vi "Finish.vi"   [LabVIEW 2020]
doc: "This VI is called just before exiting. It is expected to close I/O refnum, save collected data, etc."
uses:
  <vilib>/Rock Robotics/WPI/Utilities/WPI_GetSetVariantRefNum.vi
types:
  T1 = typedef "WPI_DigitalOutputDevRef.ctl" = cluster{"DIO Channel":T2, "DevStatus":errorcluster}
  T2 = typedef "FPGA_DIOChannel.ctl" = enum8{"DIO 0", "DIO 1", "DIO 2", "DIO 3", "DIO 4", "DIO 5", "DIO 6", "DIO 7", "DIO 8", "DIO 9", "DIO MXP 0", "DIO MXP 1", "DIO MXP 2", "DIO MXP 3", "DIO MXP 4", "DIO MXP 5", "DIO MXP 6", "DIO MXP 7", "DIO MXP 8", "DIO MXP 9", "DIO MXP 10", "DIO MXP 11", "DIO MXP 12", "DIO MXP 13", "DIO MXP 14", "DIO MXP 15", "SPI Port CS1", "SPI Port CS2", "SPI Port CS3", "SPI Port MISO", "SPI Port MOSI", "Invalid"}
  T3 = typedef "WPI_MotorControlDeviceRef.ctl" = cluster{"DeviceStatus":errorcluster, "Type":T4, "PWM":cluster{"PWM Channel":T5, "DeadBand":T6}, "CAN":cluster{"Device Number":u8, "SetOutput VI Ref":variant, "GetOutput VI Ref":variant, "Enable VI Ref":variant, "Disable VI Ref":variant, "Data":variant}, "Invert":bool, "DIO PWM":cluster{"PWM \"Enable\" Channel":T5, "DIOChannel":T2, "PWM Rate":dbl}}
  T4 = typedef "WPI_MotorControlType.ctl" = enum16{"PWM", "CAN", "DIO PWM"}
  T5 = typedef "FPGA_DIOPWMChannel.ctl" = enum8{"PWM 0", "PWM 1", "PWM 2", "PWM 3", "PWM 4", "PWM 5", "PWM 6", "PWM 7", "PWM 8", "PWM 9", "PWM MXP 0", "PWM MXP 1", "PWM MXP 2", "PWM MXP 3", "PWM MXP 4", "PWM MXP 5", "PWM MXP 6", "PWM MXP 7", "PWM MXP 8", "PWM MXP 9", "Invalid"}
  T6 = typedef "WPI_PWMDeadband.ctl" = cluster{"Name":string, "maxPositivePwm":i32, "minPositivePwm":i32, "centerPwm":i32, "maxNegativePwm":i32, "minNegativePwm":i32, "angularRange":u16}
  T7 = typedef "WPI_JoystickDevRef.ctl" = cluster{"Device":T8}
  T8 = typedef "WPI_JoystickDeviceEnum.ctl" = enum16{"USB 0", "USB 1", "USB 2", "USB 3", "USB 4", "USB 5"}
  T9 = typedef "WPI_SolenoidDevRef.ctl" = cluster{"DevStatus":errorcluster, "Pneumatics Control Module":u8, "Forward Solenoid Channel":T10, "Reverse Solenoid Channel":T10}
  T10 = typedef "WPI_SolenoidChannel.ctl" = enum8{"Solenoid 0", "Solenoid 1", "Solenoid 2", "Solenoid 3", "Solenoid 4", "Solenoid 5", "Solenoid 6", "Solenoid 7", "Solenoid 8", "Solenoid 9", "Solenoid 10", "Solenoid 11", "Solenoid 12", "Solenoid 13", "Solenoid 14", "Solenoid 15", "Invalid"}
  T11 = typedef "Color Sensor V3 DevRef.ctl" = cluster{"I2CDevRef":T12}
  T12 = typedef "WPI_I2CDevRef.ctl" = cluster{"DevStatus":errorcluster, "Device Address":u8, "Handle":i32, "I2C Bus":T13}
  T13 = typedef "i2c_bus.ctl" = enum16{"I2C On-Board", "I2C MXP", "Invalid"}
  T14 = typedef "WPI_SwitchDevRef.ctl" = cluster{"DevStatus":errorcluster, "DIO Channel":T2, "CntIndex":T15, "Normally Closed":bool}
  T15 = typedef "FPGA_CounterCtrSystemIndex.ctl" = enum8{"Ctr 0", "Ctr 1", "Ctr 2", "Ctr 3", "Ctr 4", "Ctr 5", "Ctr 6", "Ctr 7", "Invalid"}
  T16 = typedef "WPI_CompressorDevRef.ctl" = cluster{"DevStatus":errorcluster, "Pneumatics Control Module":u8}
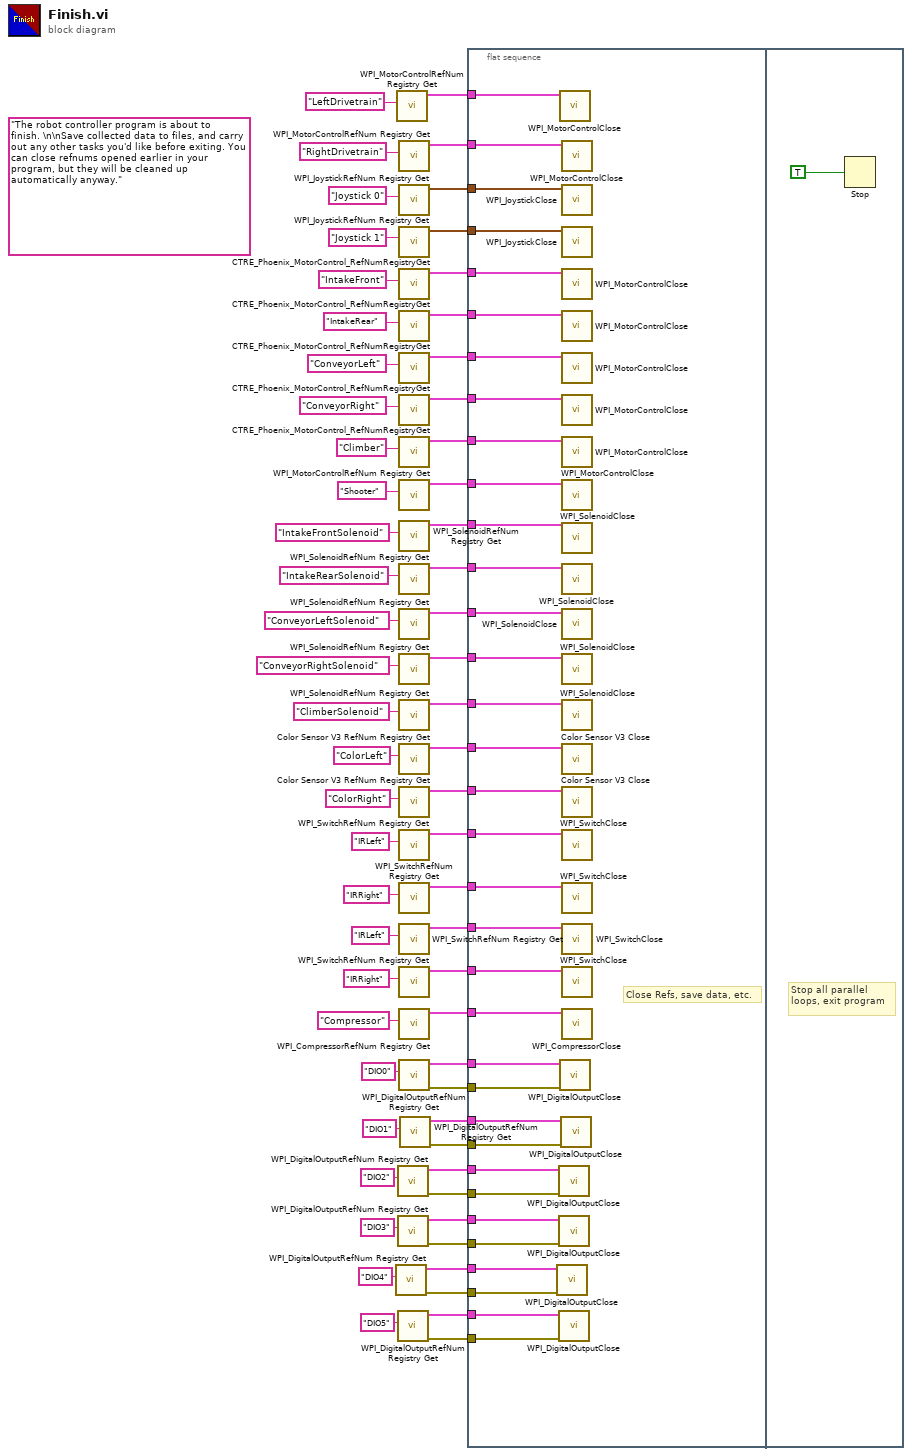
[diagram p0: block diagram]
diagram:
  (unwired) "The robot controller program is about to finish. \n\nSave collected data to files, and carry out any other tasks you'd like before exiting. You can close refnums opened earlier in your program, but they will be cleaned up automatically anyway."
  n1 = call <vilib>:"WPI_DigitalOutputRefNum Registry Get.vi"("refnum name"="DIO4") -> ("error out"=w11:errorcluster, "DigitalOutputDevRef"=w12:T1)  [unwired: 9 in]
  n2 = call <vilib>:"WPI_MotorControlRefNum Registry Get.vi"("refnum name"="LeftDrivetrain") -> ("MotorControlDevRef"=w24:T3)  [unwired: 9 in, 1 out]
  n3 = call <vilib>:"WPI_DigitalOutputRefNum Registry Get.vi"("refnum name"="DIO2") -> ("error out"=w14:errorcluster, "DigitalOutputDevRef"=w13:T1)  [unwired: 9 in]
  n4 = call <vilib>:"WPI_DigitalOutputRefNum Registry Get.vi"("refnum name"="DIO3") -> ("error out"=w8:errorcluster, "DigitalOutputDevRef"=w7:T1)  [unwired: 9 in]
  n5 = call <vilib>:"WPI_DigitalOutputRefNum Registry Get.vi"("refnum name"="DIO5") -> ("error out"=w5:errorcluster, "DigitalOutputDevRef"=w4:T1)  [unwired: 9 in]
  n6 = call <vilib>:"WPI_MotorControlRefNum Registry Get.vi"("refnum name"="RightDrivetrain") -> ("MotorControlDevRef"=w25:T3)  [unwired: 9 in, 1 out]
  n7 = call <vilib>:"WPI_JoystickRefNum Registry Get.vi"("refnum name"="Joystick 0") -> ("JoystickDevRef"=w61:T7)  [unwired: 1 in, 9 out]
  n8 = call <vilib>:"WPI_JoystickRefNum Registry Get.vi"("refnum name"="Joystick 1") -> ("JoystickDevRef"=w59:T7)  [unwired: 1 in, 9 out]
  n9 = call <vilib>:"CTRE_Phoenix_MotorControl_RefNumRegistryGet.vi"("refnum name"="IntakeFront") -> ("PhoenixMotorControlDevRef"=w58:T3)  [unwired: 9 in, 1 out]
  n10 = call <vilib>:"CTRE_Phoenix_MotorControl_RefNumRegistryGet.vi"("refnum name"="IntakeRear") -> ("PhoenixMotorControlDevRef"=w55:T3)  [unwired: 9 in, 1 out]
  n11 = call <vilib>:"CTRE_Phoenix_MotorControl_RefNumRegistryGet.vi"("refnum name"="ConveyorLeft") -> ("PhoenixMotorControlDevRef"=w51:T3)  [unwired: 9 in, 1 out]
  n12 = call <vilib>:"CTRE_Phoenix_MotorControl_RefNumRegistryGet.vi"("refnum name"="ConveyorRight") -> ("PhoenixMotorControlDevRef"=w50:T3)  [unwired: 9 in, 1 out]
  n13 = call <vilib>:"CTRE_Phoenix_MotorControl_RefNumRegistryGet.vi"("refnum name"="Climber") -> ("PhoenixMotorControlDevRef"=w49:T3)  [unwired: 9 in, 1 out]
  n14 = call <vilib>:"WPI_MotorControlRefNum Registry Get.vi"("refnum name"="Shooter") -> ("MotorControlDevRef"=w48:T3)  [unwired: 9 in, 1 out]
  n15 = call <vilib>:"WPI_SolenoidRefNum Registry Get.vi"("refnum name"="IntakeFrontSolenoid") -> ("SolenoidDevRef"=w43:T9)  [unwired: 9 in, 1 out]
  n16 = call <vilib>:"WPI_SolenoidRefNum Registry Get.vi"("refnum name"="IntakeRearSolenoid") -> ("SolenoidDevRef"=w33:T9)  [unwired: 9 in, 1 out]
  n17 = call <vilib>:"WPI_SolenoidRefNum Registry Get.vi"("refnum name"="ConveyorLeftSolenoid") -> ("SolenoidDevRef"=w42:T9)  [unwired: 9 in, 1 out]
  n18 = call <vilib>:"WPI_SolenoidRefNum Registry Get.vi"("refnum name"="ConveyorRightSolenoid") -> ("SolenoidDevRef"=w41:T9)  [unwired: 9 in, 1 out]
  n19 = call <vilib>:"WPI_SolenoidRefNum Registry Get.vi"("refnum name"="ClimberSolenoid") -> ("SolenoidDevRef"=w40:T9)  [unwired: 9 in, 1 out]
  n20 = call <vilib>:"Color Sensor V3 RefNum Registry Get.vi"("refnum name"="ColorLeft") -> ("ColorSensorDevRef"=w38:T11)  [unwired: 9 in, 1 out]
  n21 = call <vilib>:"Color Sensor V3 RefNum Registry Get.vi"("refnum name"="ColorRight") -> ("ColorSensorDevRef"=w37:T11)  [unwired: 9 in, 1 out]
  n22 = call <vilib>:"WPI_SwitchRefNum Registry Get.vi"("refnum name"="IRLeft") -> ("SwitchDevRef"=w32:T14)  [unwired: 9 in, 1 out]
  n23 = call <vilib>:"WPI_SwitchRefNum Registry Get.vi"("refnum name"="IRRight") -> ("SwitchDevRef"=w31:T14)  [unwired: 9 in, 1 out]
  n24 = call <vilib>:"WPI_SwitchRefNum Registry Get.vi"("refnum name"="IRLeft") -> ("SwitchDevRef"=w20:T14)  [unwired: 9 in, 1 out]
  n25 = call <vilib>:"WPI_SwitchRefNum Registry Get.vi"("refnum name"="IRRight") -> ("SwitchDevRef"=w19:T14)  [unwired: 9 in, 1 out]
  n26 = call <vilib>:"WPI_CompressorRefNum Registry Get.vi"("refnum name"="Compressor") -> ("CompressorDevRef"=w28:T16)  [unwired: 9 in, 1 out]
  n27 = call <vilib>:"WPI_DigitalOutputRefNum Registry Get.vi"("refnum name"="DIO0") -> ("error out"=w2:errorcluster, "DigitalOutputDevRef"=w1:T1)  [unwired: 9 in]
  n28 = call <vilib>:"WPI_DigitalOutputRefNum Registry Get.vi"("refnum name"="DIO1") -> ("error out"=w17:errorcluster, "DigitalOutputDevRef"=w18:T1)  [unwired: 9 in]
  n29 = flat-sequence {
    tunnel: w61 -> [w96]
    tunnel: w59 -> [w95]
    tunnel: w58 -> [w94]
    tunnel: w55 -> [w93]
    tunnel: w51 -> [w92]
    tunnel: w50 -> [w91]
    tunnel: w49 -> [w90]
    tunnel: w48 -> [w89]
    tunnel: w43 -> [w88]
    tunnel: w42 -> [w87]
    tunnel: w41 -> [w86]
    tunnel: w40 -> [w85]
    tunnel: w38 -> [w84]
    tunnel: w37 -> [w83]
    tunnel: w33 -> [w82]
    tunnel: w32 -> [w81]
    tunnel: w31 -> [w80]
    tunnel: w28 -> [w79]
    tunnel: w25 -> [w78]
    tunnel: w24 -> [w77]
    tunnel: w20 -> [w76]
    tunnel: w19 -> [w75]
    tunnel: w18 -> [w74]
    tunnel: w17 -> [w73]
    tunnel: w13 -> [w71]
    tunnel: w14 -> [w72]
    tunnel: w7 -> [w67]
    tunnel: w8 -> [w68]
    tunnel: w12 -> [w70]
    tunnel: w11 -> [w69]
    tunnel: w4 -> [w65]
    tunnel: w5 -> [w66]
    tunnel: w1 -> [w63]
    tunnel: w2 -> [w64]
    frame #0 {
      # "Close Refs, save data, etc."
      n30 = call <vilib>:"WPI_DigitalOutputClose.vi"("error in (no error)"=w69, "DigitalOutputDevRef"=w70) -> ()  [unwired: 9 in, 1 out]
      n31 = call <vilib>:"WPI_DigitalOutputClose.vi"("error in (no error)"=w72, "DigitalOutputDevRef"=w71) -> ()  [unwired: 9 in, 1 out]
      n32 = call <vilib>:"WPI_DigitalOutputClose.vi"("error in (no error)"=w68, "DigitalOutputDevRef"=w67) -> ()  [unwired: 9 in, 1 out]
      n33 = call <vilib>:"WPI_DigitalOutputClose.vi"("error in (no error)"=w66, "DigitalOutputDevRef"=w65) -> ()  [unwired: 9 in, 1 out]
      n34 = call <vilib>:"WPI_MotorControlClose.vi"("MotorControlDevRef"=w77) -> ()  [unwired: 10 in, 1 out]
      n35 = call <vilib>:"WPI_DigitalOutputClose.vi"("error in (no error)"=w64, "DigitalOutputDevRef"=w63) -> ()  [unwired: 9 in, 1 out]
      n36 = call <vilib>:"WPI_DigitalOutputClose.vi"("error in (no error)"=w73, "DigitalOutputDevRef"=w74) -> ()  [unwired: 9 in, 1 out]
      n37 = call <vilib>:"WPI_MotorControlClose.vi"("MotorControlDevRef"=w78) -> ()  [unwired: 10 in, 1 out]
      n38 = call <vilib>:"WPI_JoystickClose.vi"("JoystickDevRef"=w96) -> ()  [unwired: 11 out]
      n39 = call <vilib>:"WPI_JoystickClose.vi"("JoystickDevRef"=w95) -> ()  [unwired: 11 out]
      n40 = call <vilib>:"WPI_MotorControlClose.vi"("MotorControlDevRef"=w94) -> ()  [unwired: 10 in, 1 out]
      n41 = call <vilib>:"WPI_MotorControlClose.vi"("MotorControlDevRef"=w93) -> ()  [unwired: 10 in, 1 out]
      n42 = call <vilib>:"WPI_MotorControlClose.vi"("MotorControlDevRef"=w92) -> ()  [unwired: 10 in, 1 out]
      n43 = call <vilib>:"WPI_MotorControlClose.vi"("MotorControlDevRef"=w91) -> ()  [unwired: 10 in, 1 out]
      n44 = call <vilib>:"WPI_MotorControlClose.vi"("MotorControlDevRef"=w90) -> ()  [unwired: 10 in, 1 out]
      n45 = call <vilib>:"WPI_MotorControlClose.vi"("MotorControlDevRef"=w89) -> ()  [unwired: 10 in, 1 out]
      n46 = call <vilib>:"WPI_SolenoidClose.vi"("SolenoidDevRef"=w88) -> ()  [unwired: 10 in, 1 out]
      n47 = call <vilib>:"WPI_SolenoidClose.vi"("SolenoidDevRef"=w82) -> ()  [unwired: 10 in, 1 out]
      n48 = call <vilib>:"WPI_SolenoidClose.vi"("SolenoidDevRef"=w87) -> ()  [unwired: 10 in, 1 out]
      n49 = call <vilib>:"WPI_SolenoidClose.vi"("SolenoidDevRef"=w86) -> ()  [unwired: 10 in, 1 out]
      n50 = call <vilib>:"WPI_SolenoidClose.vi"("SolenoidDevRef"=w85) -> ()  [unwired: 10 in, 1 out]
      n51 = call <vilib>:"Color Sensor V3 Close.vi"("ColorSensorDevRef in"=w84) -> ()  [unwired: 10 in, 1 out]
      n52 = call <vilib>:"Color Sensor V3 Close.vi"("ColorSensorDevRef in"=w83) -> ()  [unwired: 10 in, 1 out]
      n53 = call <vilib>:"WPI_SwitchClose.vi"("SwitchDevRef"=w81) -> ()  [unwired: 10 in, 1 out]
      n54 = call <vilib>:"WPI_SwitchClose.vi"("SwitchDevRef"=w80) -> ()  [unwired: 10 in, 1 out]
      n55 = call <vilib>:"WPI_SwitchClose.vi"("SwitchDevRef"=w76) -> ()  [unwired: 10 in, 1 out]
      n56 = call <vilib>:"WPI_SwitchClose.vi"("SwitchDevRef"=w75) -> ()  [unwired: 10 in, 1 out]
      n57 = call <vilib>:"WPI_CompressorClose.vi"("CompressorDevRef"=w79) -> ()  [unwired: 10 in, 1 out]
    }
    frame #1 {
      # "Stop all parallel\nloops, exit program"
      n58 = Stop(stop? (T)=TRUE ("Quit")) -> ()
    }
  }
